vi "QMH_Class Temp.vi"() -> ()   [LabVIEW 2018, in "QMH_Class.lvlib"]
uses:
  QMH_Class.lvlib
  Device/TempChamber/TempChamber Weiss/TempChamber Weiss.lvclass
  Device/TempChamber/TempChamber Sim/TempChamber Sim.lvclass
  E:/0 File/GITSync/DynoToolPlus/0 LabviewCode/0 Support/Message Queue_Class/Device/TempChamber/TempChamber Interface/TempChamber Interface.lvclass
  Class/Execute_class/Execute.lvclass/Execute.ctl
  Class/Message_class/InterfaceMessage/Interface Message.lvclass
  Class/Message_class/SetPowerMessage/SetPower Message.lvclass
  Class/Message_class/StopMessage/Stop Message.lvclass
  Class/Message_class/SetTempMessage/SetTemp Message.lvclass
  Class/Execute_class/Execute.lvclass
panel:
  in  "SetTemp":bool
  in  "Temp":dbl
  in  "Humid":dbl
  in  "Exit":bool
  in  "SetPower":bool
  in  "PowerType":enum16{"Itech", "Keysight"}(ring)
  in  "Volt":dbl
  out "SoftVersion":string
  out "User":string
  out "Log":string
  out "Status":bool
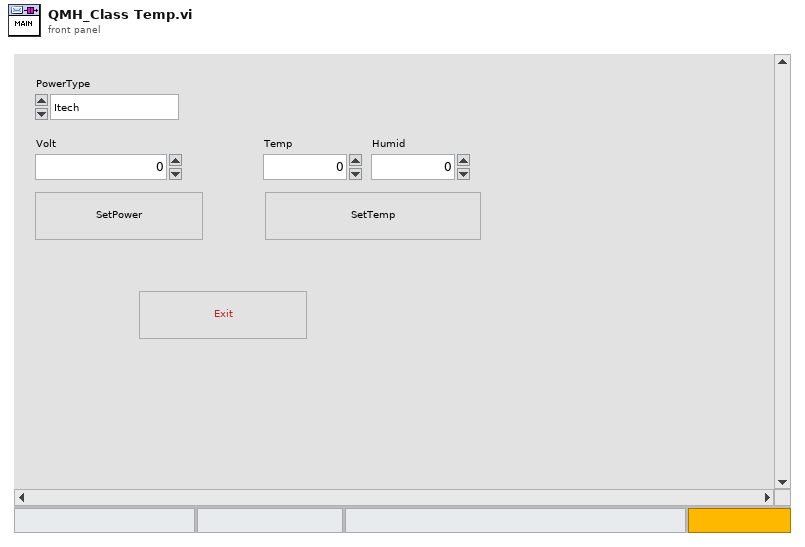
[diagram p1: front panel]
types:
  T1 = cluster{"Event":cluster{"Stop":refnum<user-event>}, "输出簇":cluster{"Status":refnum<vi>, "Log":refnum<vi>, "User":refnum<vi>, "SoftVersion":refnum<vi>}}
  T2 = cluster{"Volt":dbl, "PowerType":enum16{"Itech", "Keysight"}}
  T3 = enum32{"invalid app kind", "Development System", "Run Time System", "Student Edition", "Embedded LabVIEW", "Evaluation", "Custom"}
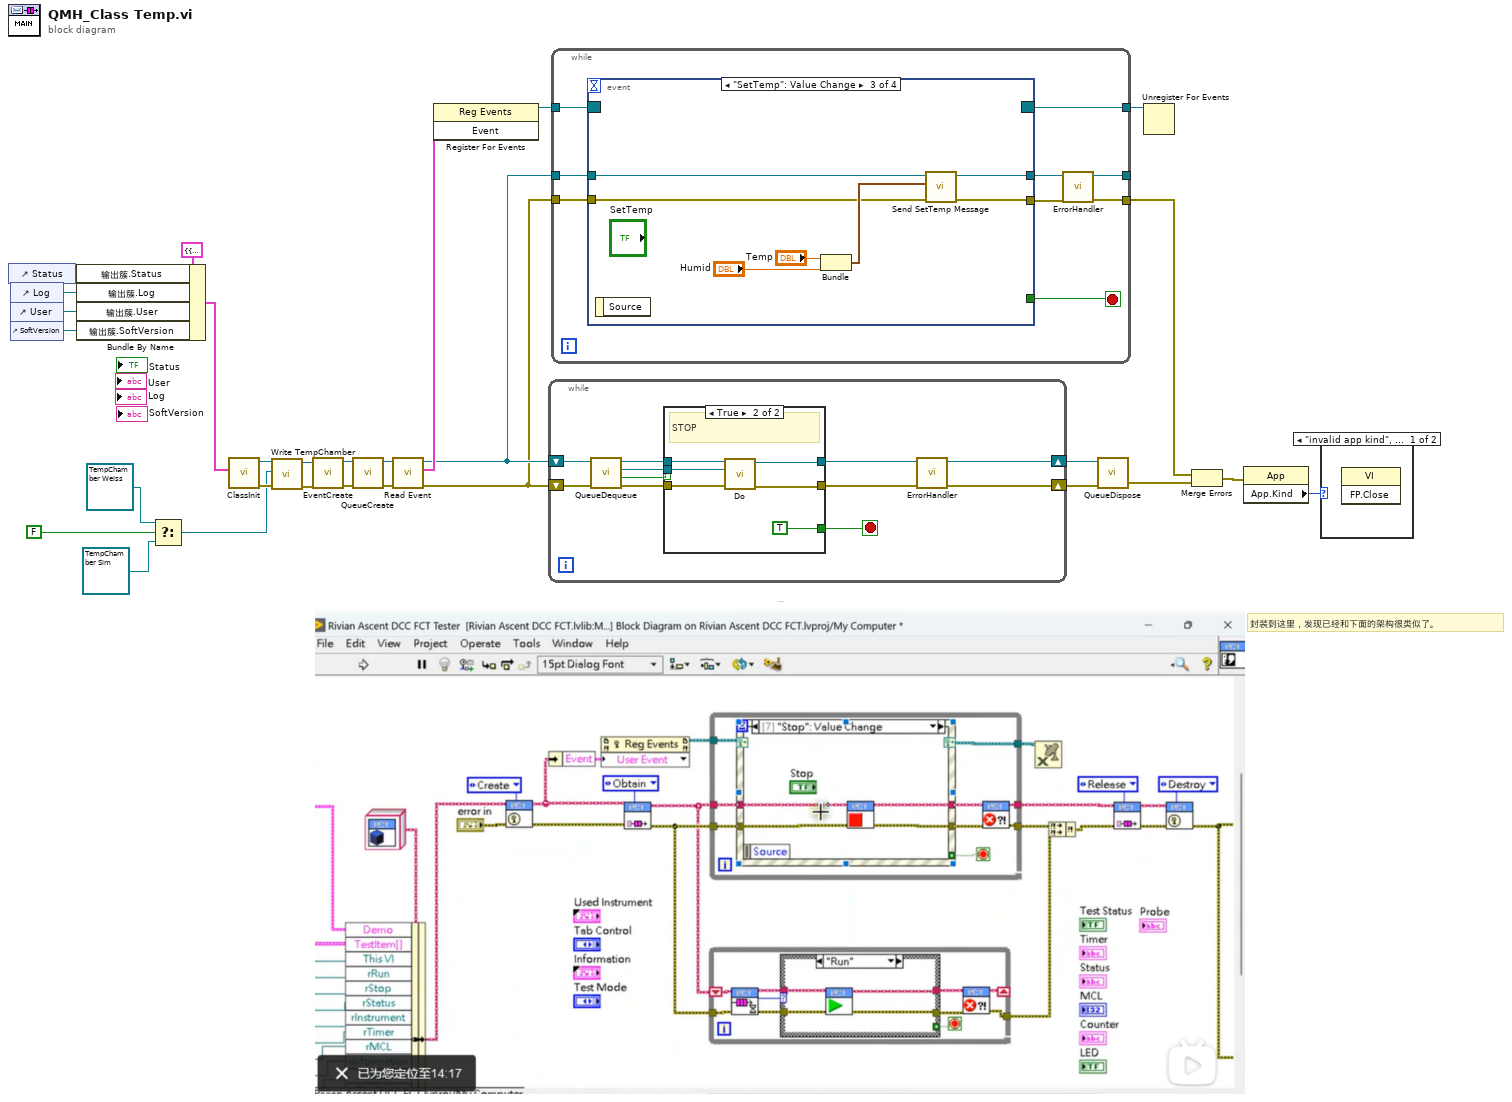
[diagram p0: block diagram]
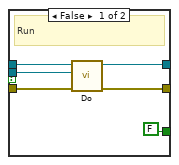
[diagram p2: hidden frame]
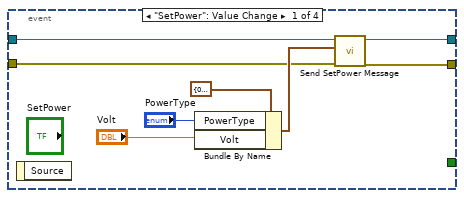
[diagram p3: hidden frame]
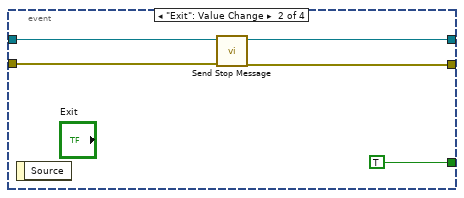
[diagram p4: hidden frame]
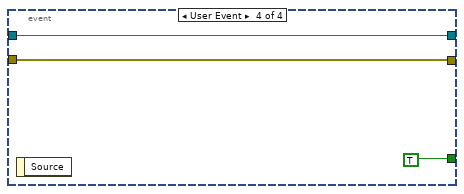
[diagram p5: hidden frame]
diagram:
  # "封装到这里，发现已经和下面的架构很类似了。"
  n1 = control-ref of="Status"() -> (w25:refnum<vi>)
  n2 = control-ref of="Log"() -> (w24:refnum<vi>)
  n3 = control-ref of="User"() -> (w23:refnum<vi>)
  n4 = control-ref of="SoftVersion"() -> (w22:refnum<vi>)
  n5 = Bundle By Name(cluster=T1 {"Event"={"Stop"=refnum}, "输出簇"={"Status"=refnum, "Log"=refnum, "User"=refnum, "SoftVersion"=refnum}} ("data"), "输出簇.Status"=w25, "输出簇.Log"=w24, "输出簇.User"=w23, "输出簇.SoftVersion"=w22) -> (w21:T1)
  n6 = Select(t=refnum<class "TempChamber Weiss.lvclass"> refnum ("QMH_Class.lvlib:Device.lvlib:TempChamber Weiss.lvclass"), s=FALSE, f=refnum<class "TempChamber Sim.lvclass"> refnum ("QMH_Class.lvlib:Device.lvlib:TempChamber Sim.lvclass")) -> (s? t:f=w2:refnum<class "TempChamber Interface.lvclass">)
  n7 = call "ClassInit.vi"("data"=w21) -> ("error out"=w5:errorcluster, "Execute"=w8:refnum<class "Execute.lvclass">)  [unwired: 9 in]
  n8 = call "Write TempChamber.vi"("error in (no error)"=w5, "QMH_Class.lvlib:Device.lvlib:TempChamber Interface.lvclass"=w2, "Execute in"=w8) -> ("error out"=w6:errorcluster, "Execute out"=w7:refnum<class "Execute.lvclass">)  [unwired: 7 in]
  n9 = call "EventCreate.vi"("error in (no error)"=w6, "Execute"=w7) -> ("error out"=w17:errorcluster, "Execute"=w16:refnum<class "Execute.lvclass">)  [unwired: 8 in]
  n10 = call "QueueCreate.vi"("error in (no error)"=w17, "Execute"=w16) -> ("error out"=w19:errorcluster, "Execute"=w20:refnum<class "Execute.lvclass">)  [unwired: 8 in]
  n11 = call "Read Event.vi"("error in (no error)"=w19, "Execute"=w20) -> ("error out"=w14:errorcluster, "Event"=w18:cluster{"Stop":refnum<user-event>}, "Execute"=w15:refnum<class "Execute.lvclass">)  [unwired: 7 in]
  n12 = register-events(w18) -> (reference out=w28:refnum<event-registration>)  [unwired: 2 in, 1 out]
  n13 = while {
    shift-right: [w39] -> w11
    shift-left: w15 -> [w35]
    shift-right: [w38] -> w12
    shift-left: w14 -> [w40]
    stop <- w30 stop-if-true
    n14 = call "QueueDequeue.vi"("error in (no error)"=w40, "Execute"=w35) -> ("error out"=w36:errorcluster, "Stop"=w31:bool, "Interface Message"=w33:refnum<class "Interface Message.lvclass">, "Execute"=w34:refnum<class "Execute.lvclass">)  [unwired: 6 in]
    n15 = case shown="True" w31 {
      tunnel: [w46 w49] -> w37
      tunnel: w36 -> [w45 w51]
      tunnel: w34 -> [w44 w52]
      tunnel: w33 -> [w43 w48]
      tunnel: [w42 w50] -> w32
      tunnel: [FALSE TRUE] -> w30
      frame False {
        # "Run"
        n16 = call-dynamic "Do.vi"("error in (no error)"=w45, "Message in"=w43, "Execute"=w44) -> ("error out"=w46:errorcluster, "Execute"=w42:refnum<class "Execute.lvclass">)  [unwired: 6 in, 1 out]
      }
      frame True {
        # "STOP"
        n17 = call-dynamic "Do.vi"("error in (no error)"=w51, "Message in"=w48, "Execute"=w52) -> ("error out"=w49:errorcluster, "Execute"=w50:refnum<class "Execute.lvclass">)  [unwired: 6 in, 1 out]
      }
    }
    n18 = call "ErrorHandler.vi"("错误输入（无错误）"=w37, "Execute输入"=w32) -> ("错误输出"=w38:errorcluster, "Execute输出"=w39:refnum<class "Execute.lvclass">)  [unwired: 8 in]
  }
  n19 = while {
    tunnel: w15 -> [w61]
    tunnel: w28 -> [w59]
    tunnel: [w58] -> w27
    tunnel: w14 -> [w57]
    tunnel: [w54] -> _
    tunnel: [w53] -> w10
    stop <- w60 stop-if-true
    n20 = event shown="[2] \"SetTemp\": Value Change" {
      selector: w59 -> [_ _ _ _]
      dyn-events: [_ _ _ _] -> w58
      timeout: _ -> [_ _ _ _]
      tunnel: w61 -> [w66 w73 w79 w83]
      tunnel: [_ TRUE _ TRUE] -> w60
      tunnel: w57 -> [w62 w72 w76 w82]
      tunnel: [w64 w71 w77 w83] -> w55
      tunnel: [w63 w70 w75 w82] -> w56
      event "SetPower": Value Change {
        n21 = event-data() -> ()  [unwired: 1 in, 1 out]
        n22 = Bundle By Name(cluster=T2 {"Volt"=0.0, "PowerType"=enum."Itech"} ("PowerData"), "PowerType"="PowerType", "Volt"="Volt") -> (w65:T2)
        n23 = call "Send SetPower Message.vi"("error in (no error)"=w62, "PowerData"=w65, "Execute"=w66) -> ("error out"=w63:errorcluster, "Execute 2"=w64:refnum<class "Execute.lvclass">)  [unwired: 7 in]
      }
      event "Exit": Value Change {
        n24 = event-data() -> ()  [unwired: 1 in, 1 out]
        n25 = call "Send Stop Message.vi"("error in (no error)"=w72, "Execute"=w73) -> ("error out"=w70:errorcluster, "Execute"=w71:refnum<class "Execute.lvclass">)  [unwired: 8 in]
      }
      event "SetTemp": Value Change {
        n26 = event-data() -> ()  [unwired: 1 in, 1 out]
        n27 = Bundle("Temp"="Temp", "Humid"="Humid") -> (w78:cluster{"Temp":dbl, "Humid":dbl})  [unwired: 1 in]
        n28 = call "Send SetTemp Message.vi"("error in (no error)"=w76, "Cluster"=w78, "Execute"=w79) -> ("error out"=w75:errorcluster, "Execute 2"=w77:refnum<class "Execute.lvclass">)  [unwired: 7 in]
      }
      event User Event {
        n29 = event-data() -> ()  [unwired: 1 in, 1 out]
      }
    }
    n30 = call "ErrorHandler.vi"("错误输入（无错误）"=w56, "Execute输入"=w55) -> ("错误输出"=w53:errorcluster, "Execute输出"=w54:refnum<class "Execute.lvclass">)  [unwired: 8 in]
  }
  n31 = call "QueueDispose.vi"("error in (no error)"=w12, "Execute"=w11) -> ("error out"=w9:errorcluster)  [unwired: 8 in, 1 out]
  n32 = Unregister For Events(event registration refnum=w27) -> ()  [unwired: 1 in, 1 out]
  n33 = Merge Errors(w10, w9) -> (w13:errorcluster)
  n34 = property class="App"(error in=w13) -> ("App.Kind"=w29:T3)  [unwired: 1 in, 2 out]
  n35 = case shown="\"invalid app kind\", Default" w29 {
    frame "invalid app kind", Default {
      n36 = invoke class="VI" method="FP.Close"() -> ()  [unwired: 3 in, 3 out]
    }
    frame "Development System" {
    }
  }
